vi "告警码字段定义.vi"(11 "告警代码":u16) -> (3 "报警":T1)   [LabVIEW 2016, in "斯坦道总氮V2.lvlib"]
uses:
  Alarm interface/Alarm interface.lvlib
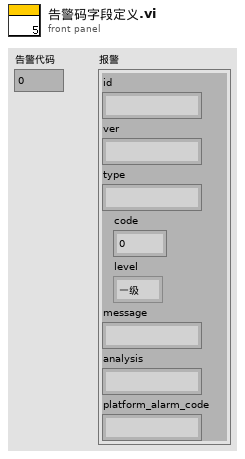
[diagram p1: front panel]
types:
  T1 = cluster{"id":string, "ver":string, "type":string, "code":u16, "level":enum16{"一级", "二级", "三级"}, "message":string, "analysis":string, "platform_alarm_code":string}
  T2 = cluster{"id":string, "ver":string, "type":enum16{"Alarm", "Fault"}, "code":u16}
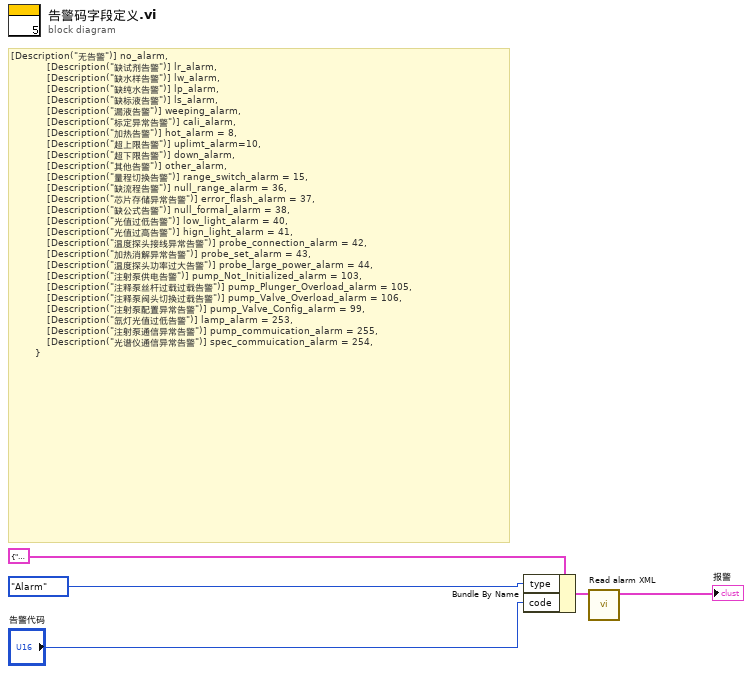
[diagram p0: block diagram]
diagram:
  # "[Description(\"无告警\")] no_alarm,\n            [Description(\"缺试剂告警\")] lr_alarm,\n            [Description(\"缺水样告警\")] lw_alarm,\n            [Description(\"缺纯水告警\")] lp_alarm,\n            [Description(\"缺标液告警\")] ls_alarm,\n            [Description(\"漏液告警\")] weeping_alarm,\n            [Description(\"标定异常告警\")] cali_alarm,\n            [Description(\"加热告警\")] hot_alarm = 8,\n            [Description(\"超上限告警\")] uplimt_alarm=10,\n            [Description(\"超下限告警\")] down_alarm,\n            [Description(\"其他告警\")] other_alarm,\n            [Description(\"量程切换告警\")] range_switch_alarm = 15,\n            [Description(\"缺流程告警\")] null_range_alarm = 36,\n            [Description(\"芯片存储异常告警\")] error_flash_alarm = 37,\n            [Description(\"缺公式告警\")] null_formal_alarm = 38,\n            [Description(\"光值过低告警\")] low_light_alarm = 40,\n            [Description(\"光值过高告警\")] hign_light_alarm = 41,\n            [Description(\"温度探头接线异常告警\")] probe_connection_alarm = 42,\n            [Description(\"加热消解异常告警\")] probe_set_alarm = 43,\n            [Description(\"温度探头功率过大告警\")] probe_large_power_alarm = 44,\n            [Description(\"注射泵供电告警\")] pump_Not_Initialized_alarm = 103,\n            [Description(\"注释泵丝杆过载过载告警\")] pump_Plunger_Overload_alarm = 105,\n            [Description(\"注释泵阀头切换过载告警\")] pump_Valve_Overload_alarm = 106,\n            [Description(\"注射泵配置异常告警\")] pump_Valve_Config_alarm = 99,\n            [Description(\"氙灯光值过低告警\")] lamp_alarm = 253,\n            [Description(\"注射泵通信异常告警\")] pump_commuication_alarm = 255,\n            [Description(\"光谱仪通信异常告警\")] spec_commuication_alarm = 254,\n        }"
  n1 = Bundle By Name(cluster=T2 {"id"="斯坦道营养盐", "ver"="A", "type"=enum."Alarm", "code"=1} ("筛选输入"), "type"=enum16{"Alarm", "Fault"}."Alarm", "code"="告警代码") -> (w4:T2)
  n2 = call "Read alarm XML.vi"("筛选输入"=w4) -> ("报警"=→"报警":T1)  [unwired: 9 in]
